vi "ConfigParseImage.vi"(8 "error in (no error)":errorcluster, 10 "Refnum in":refnum<k20>) -> (0 "error out":errorcluster, 2 "Array out":string[][](array[string]))   [LabVIEW 2018]
uses:
  <vilib>/xml/NI_XML.lvlib
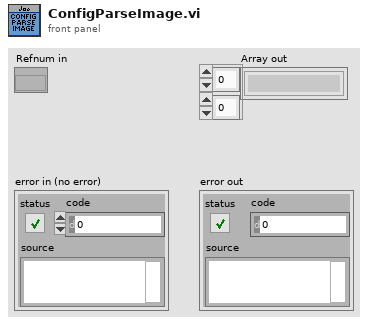
[diagram p1: front panel]
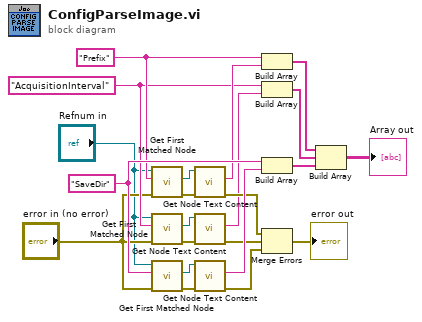
[diagram p0: block diagram]
diagram:
  w19 = "SaveDir" ("XPath expression")
  w11 = "AcquisitionInterval" ("XPath expression")
  w12 = "Prefix" ("XPath expression")
  n1 = call <vilib>:"Get First Matched Node.vi"("error in (no error)"="error in (no error)", "XPath expression"=w12, "node in"="Refnum in") -> ("error out"=w5:errorcluster, "node result"=w4:refnum<k20>)  [unwired: 6 in, 1 out]
  n2 = call <vilib>:"Get First Matched Node.vi"("error in (no error)"="error in (no error)", "XPath expression"=w11, "node in"="Refnum in") -> ("error out"=w7:errorcluster, "node result"=w6:refnum<k20>)  [unwired: 6 in, 1 out]
  n3 = call <vilib>:"Get First Matched Node.vi"("error in (no error)"="error in (no error)", "XPath expression"=w19, "node in"="Refnum in") -> ("error out"=w9:errorcluster, "node result"=w8:refnum<k20>)  [unwired: 6 in, 1 out]
  n4 = call <vilib>:"Get Node Text Content.vi"("error in (no error)"=w5, "node in"=w4) -> ("error out"=w16:errorcluster, "node text"=w13:string)  [unwired: 7 in, 1 out]
  n5 = call <vilib>:"Get Node Text Content.vi"("error in (no error)"=w7, "node in"=w6) -> ("error out"=w17:errorcluster, "node text"=w10:string)  [unwired: 7 in, 1 out]
  n6 = call <vilib>:"Get Node Text Content.vi"("error in (no error)"=w9, "node in"=w8) -> ("error out"=w18:errorcluster, "node text"=w20:string)  [unwired: 7 in, 1 out]
  n7 = Build Array(w12, w13) -> (w14:string[])
  n8 = Build Array(w11, w10) -> (w15:string[])
  n9 = Build Array(w19, w20) -> (w21:string[])
  n10 = Merge Errors(w16, w17, w18) -> (→"error out":errorcluster)
  n11 = Build Array(w14, w15, w21) -> (→"Array out":string[][])
